vi "GUI.vi"() -> ()   [LabVIEW 2013]
uses:
  C:/Program Files/Newport/Piezo Motion Control/Newport AG-UC2-UC8 Applet/Samples/LabVIEW 2009/AgilisCmdLib.dll
  Program Files/Newport/Piezo Motion Control/Newport AG-UC2-UC8 Applet/Samples/LabVIEW 2009/AgilisCmdLib.dll
panel:
  out "currentPosition":dbl
  in  "Position":dbl format="%.6f"
  in  "Center Device":bool
  out "Messages":string
  out "Last Calibration":string
  out "Average step size in reverse direction (mm)":dbl
  out "Average step size in forward direction (mm)":dbl
  in  "travelRange":i32
  in  "Step Size (nm)":i32=1 min=1 max=50 step=1
  out "reference":refnum<k24>
  out "axis":i32
  in  "Select Axis Number":string(combo)
  in  "Stop Device and Terminate Program":bool
  in  "Select COM Port":string(combo)
  in  "Calibrate":bool
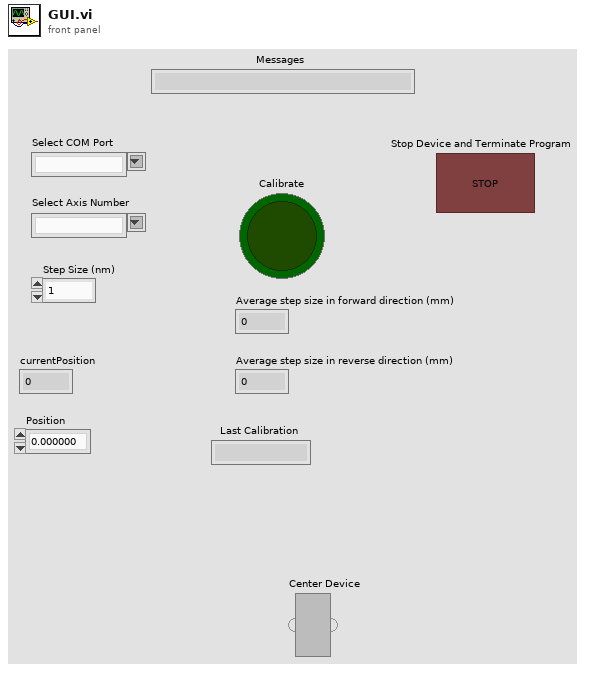
[diagram p1: front panel]
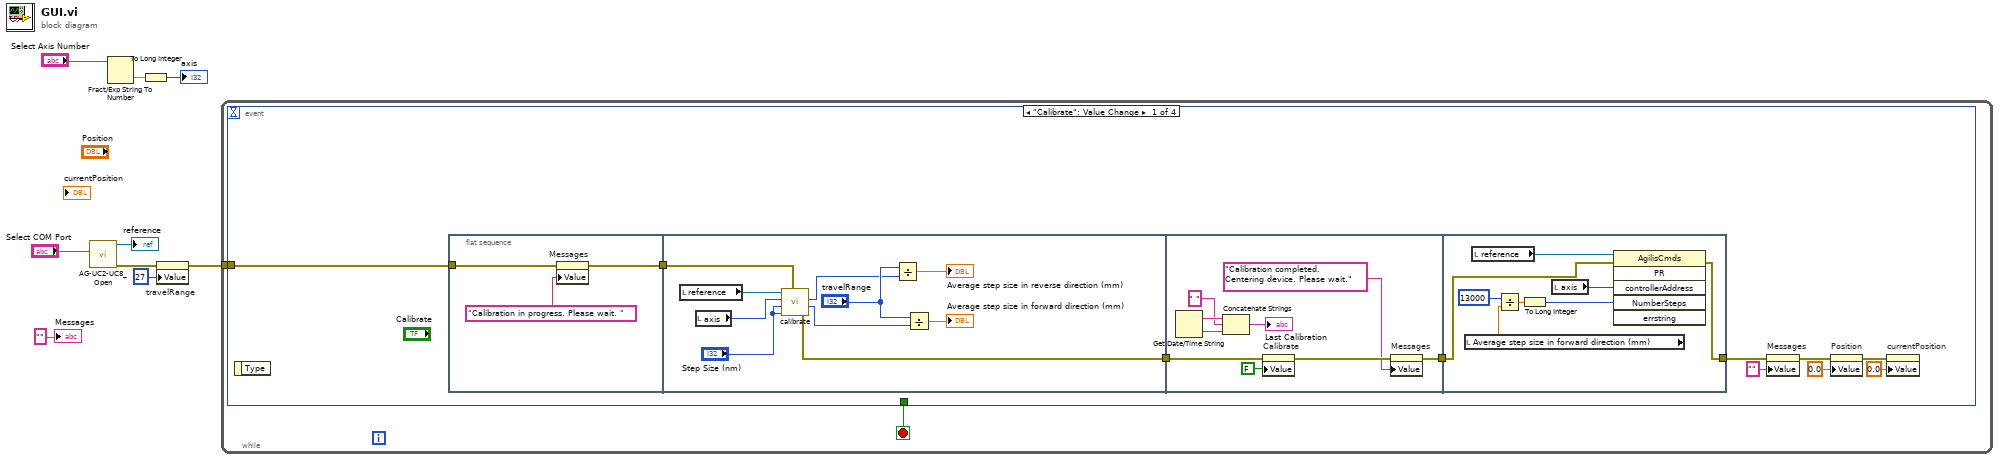
[diagram p0: block diagram]
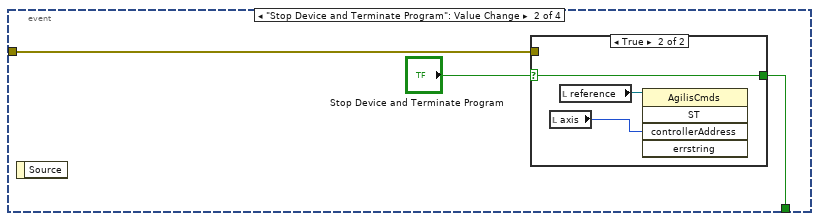
[diagram p2: hidden frame]
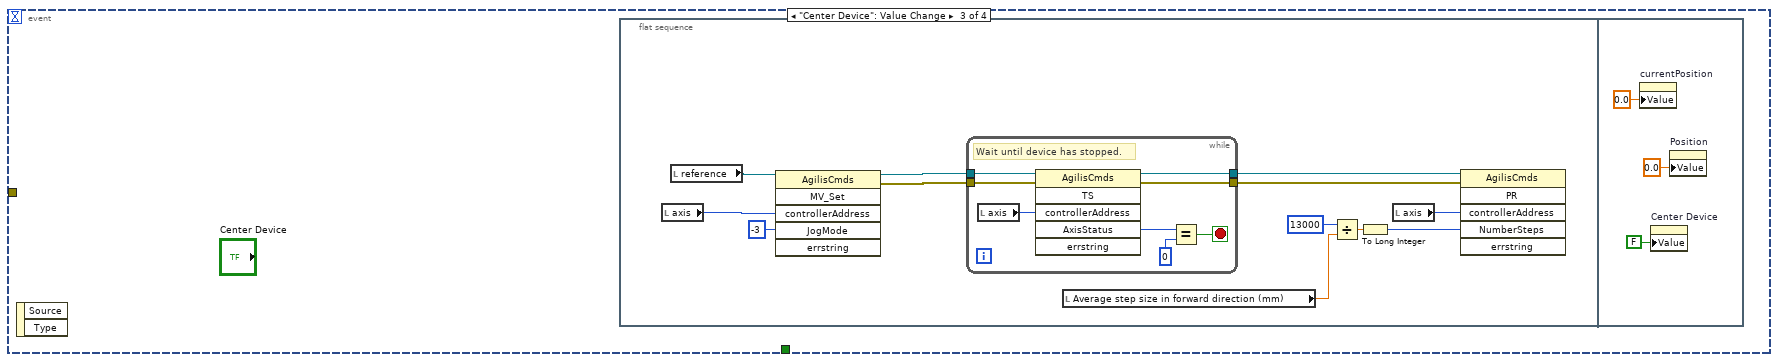
[diagram p4: hidden frame]
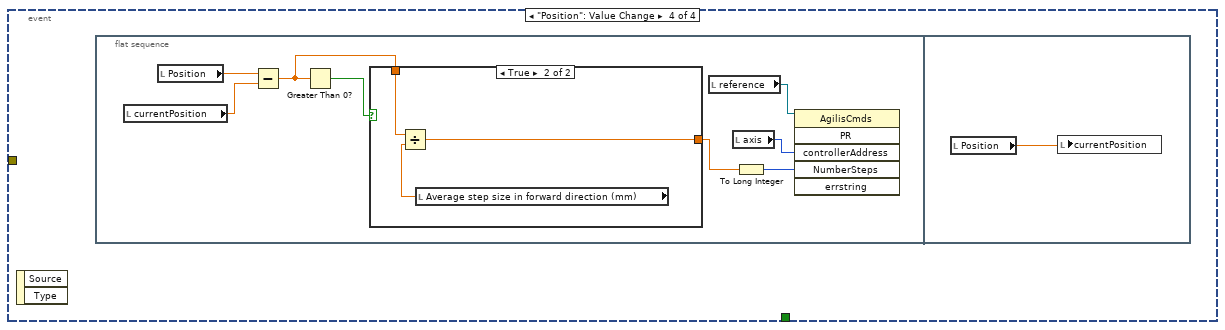
[diagram p5: hidden frame]
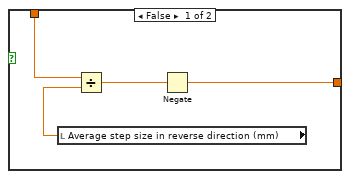
[diagram p6: hidden frame]
diagram:
  n1 = call "AG-UC2-UC8_Open.vi"("Instrument Key IN"="Select COM Port") -> ("error out"=w4:errorcluster, "AG-UC2-UC8 Reference"=→"reference":refnum<k24>)  [unwired: 3 in, 2 out]
  n2 = Fract/Exp String To Number(string="Select Axis Number") -> (number=w7:dbl)  [unwired: 3 in, 1 out]
  n3 = To Long Integer(number=w7) -> (32bit integer=→"axis":i32)
  n4 = property on="travelRange" class="DigNum (strict)"(error in=w4, "Value"=i16 27 ("Travel Range (mm)")) -> (error out=w2:errorcluster)  [unwired: 1 in, 1 out]
  n5 = while {
    tunnel: w2 -> [w10]
    stop <- w11 stop-if-true
    n6 = event shown="[0] \"Calibrate\": Value Change" {
      selector: _ -> [_ _ _ _]
      dyn-events: _ -> [_ _ _ _]
      timeout: _ -> [_ _ _ _]
      tunnel: [_ w53 _ _] -> w11
      tunnel: w10 -> [w21 w52 _ _]
      event "Calibrate": Value Change {
        n7 = event-data() -> ()  [unwired: 1 in, 1 out]
        n8 = flat-sequence {
          tunnel: w21 -> [w24]
          tunnel: [w23] -> w19
          tunnel: [w28] -> w20
          tunnel: w19 -> [w34]
          tunnel: w20 -> [w39]
          tunnel: [w36] -> w18
          tunnel: w18 -> [w45]
          tunnel: [w44] -> w16
          frame #0 {
            n9 = property on="Messages" class="Str"(error in=w24, "Value"="Calibration in progress. Please wait. " ("message")) -> (error out=w23:errorcluster)  [unwired: 1 in, 1 out]
          }
          frame #1 {
            n10 = local read "reference"() -> (w33:refnum<k24>)
            n11 = local read "axis"() -> (w32:i32)
            n12 = call "calibrate.vi"("errorIn"=w34, "reverseStepSize"="Step Size (nm)", "forwardStepSize"="Step Size (nm)", "axis"=w32, "referenceIn"=w33) -> ("errorOut"=w28:errorcluster, "nForwardSteps"=w26:i32, "nReverseSteps"=w25:i32)  [unwired: 1 out]
            n13 = Divide(x="travelRange", y=w25) -> (x/y=→"Average step size in reverse direction (mm)":dbl)
            n14 = Divide(x="travelRange", y=w26) -> (x/y=→"Average step size in forward direction (mm)":dbl)
          }
          frame #2 {
            n15 = Get Date/Time String() -> (date string=w43:string, time string=w42:string)  [unwired: 3 in]
            n16 = Concatenate Strings(w43, " " ("string"), w42) -> (→"Last Calibration":string)
            n17 = property on="Calibrate" class="Bool (strict)"(error in=w39, "Value"=FALSE ("Calibrate")) -> (error out=w37:errorcluster)  [unwired: 1 in, 1 out]
            n18 = property on="Messages" class="Str"(error in=w37, "Value"="Calibration completed. Centering device. Please wait." ("Messages")) -> (error out=w36:errorcluster)  [unwired: 1 in, 1 out]
          }
          frame #3 {
            n19 = local read "Average step size in forward direction (mm)"() -> (w50:dbl)
            n20 = local read "reference"() -> (w48:refnum<k24>)
            n21 = Divide(x=13000, y=w50) -> (x/y=w49:dbl)
            n22 = To Long Integer(number=w49) -> (32bit integer=w46:i32)
            n23 = local read "axis"() -> (w47:i32)
            n24 = invoke class="AgilisCmds" method="PR"(reference=w48, error in=w45, "controllerAddress"=w47, "NumberSteps"=w46) -> (error out=w44:errorcluster)  [unwired: 2 in, 5 out]
          }
        }
        n25 = property on="Messages" class="Str"(error in=w16, "Value"="" ("Messages")) -> (error out=w15:errorcluster)  [unwired: 1 in, 1 out]
        n26 = property on="Position" class="DigNum (strict)"(error in=w15, "Value"=0.0 ("Numeric")) -> (error out=w13:errorcluster)  [unwired: 1 in, 1 out]
        n27 = property on="currentPosition" class="DigNum (strict)"(error in=w13, "Value"=0.0 ("currentPosition")) -> ()  [unwired: 1 in, 2 out]
      }
      event "Stop Device and Terminate Program": Value Change {
        n28 = event-data() -> ()  [unwired: 1 in, 1 out]
        n29 = case shown="True" "Stop Device and Terminate Program" {
          selector: "Stop Device and Terminate Program" -> [w55 w57]
          tunnel: [w55 w57] -> w53
          tunnel: w52 -> [_ _]
          frame False {
          }
          frame True {
            n30 = local read "axis"() -> (w58:i32)
            n31 = local read "reference"() -> (w56:refnum<k24>)
            n32 = invoke class="AgilisCmds" method="ST"(reference=w56, "controllerAddress"=w58) -> ()  [unwired: 3 in, 5 out]
          }
        }
      }
      event "Center Device": Value Change {
        n33 = event-data() -> ()  [unwired: 1 in, 2 out]
        n34 = flat-sequence {
          frame #0 {
            n35 = local read "axis"() -> (w66:i32)
            n36 = local read "reference"() -> (w63:refnum<k24>)
            n37 = invoke class="AgilisCmds" method="MV_Set"(reference=w63, "controllerAddress"=w66, "JogMode"=-3) -> (reference out=w60:refnum<k24>, error out=w59:errorcluster)  [unwired: 3 in, 4 out]
            n38 = while {
              tunnel: [w75] -> w62
              tunnel: [w74] -> w61
              tunnel: w60 -> [w73]
              tunnel: w59 -> [w72]
              stop <- w76 stop-if-true
              # "Wait until device has stopped."
              n39 = local read "axis"() -> (w71:i32)
              n40 = invoke class="AgilisCmds" method="TS"(reference=w73, error in=w72, "controllerAddress"=w71) -> (reference out=w75:refnum<k24>, error out=w74:errorcluster, "AxisStatus"=w78:i32)  [unwired: 3 in, 3 out]
              n41 = Equal?(x=w78, y=0) -> (x = y?=w76:bool)
            }
            n42 = local read "Average step size in forward direction (mm)"() -> (w64:dbl)
            n43 = Divide(x=13000, y=w64) -> (x/y=w68:dbl)
            n44 = To Long Integer(number=w68) -> (32bit integer=w67:i32)
            n45 = local read "axis"() -> (w65:i32)
            n46 = invoke class="AgilisCmds" method="PR"(reference=w62, error in=w61, "controllerAddress"=w65, "NumberSteps"=w67) -> ()  [unwired: 2 in, 6 out]
          }
          frame #1 {
            n47 = property on="currentPosition" class="DigNum (strict)"("Value"=0.0 ("currentPosition")) -> ()  [unwired: 2 in, 2 out]
            n48 = property on="Center Device" class="Bool (strict)"("Value"=FALSE ("Center Device 2")) -> ()  [unwired: 2 in, 2 out]
            n49 = property on="Position" class="DigNum (strict)"("Value"=0.0 ("Numeric")) -> ()  [unwired: 2 in, 2 out]
          }
        }
      }
      event "Position": Value Change {
        n50 = event-data() -> ()  [unwired: 1 in, 2 out]
        n51 = flat-sequence {
          frame #0 {
            n52 = local read "currentPosition"() -> (w88:dbl)
            n53 = local read "Position"() -> (w89:dbl)
            n54 = Subtract(x=w89, y=w88) -> (x-y=w87:dbl)
            n55 = Greater Than 0?(x=w87) -> (x > 0?=w86:bool)
            n56 = case shown="True" w86 {
              tunnel: w87 -> [w93 w96]
              tunnel: [w90 w94] -> w85
              frame False {
                n57 = local read "Average step size in reverse direction (mm)"() -> (w92:dbl)
                n58 = Divide(x=w93, y=w92) -> (x/y=w91:dbl)
                n59 = Negate(x=w91) -> (-x=w90:dbl)
              }
              frame True {
                n60 = local read "Average step size in forward direction (mm)"() -> (w95:dbl)
                n61 = Divide(x=w96, y=w95) -> (x/y=w94:dbl)
              }
            }
            n62 = local read "reference"() -> (w83:refnum<k24>)
            n63 = local read "axis"() -> (w82:i32)
            n64 = To Long Integer(number=w85) -> (32bit integer=w84:i32)
            n65 = invoke class="AgilisCmds" method="PR"(reference=w83, "controllerAddress"=w82, "NumberSteps"=w84) -> ()  [unwired: 3 in, 6 out]
          }
          frame #1 {
            n66 = local read "Position"() -> (w97:dbl)
            n67 = local write "currentPosition"(w97) -> ()
          }
        }
      }
    }
  }
  "Messages" <- "" ("Messages")
